vi "sub_DC Power End.vi"(8 "错误输入（无错误）":errorcluster, 10 "instrument handle out":refnum<k15>, 11 "IVI引用句柄输入":refnum<k15>) -> ()   [LabVIEW 2015]
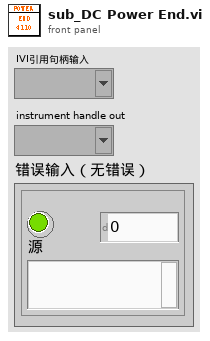
[diagram p1: front panel]
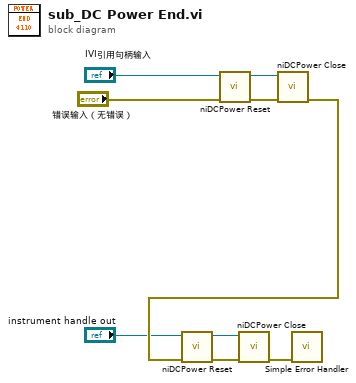
[diagram p0: block diagram]
diagram:
  n1 = call <instrlib>:"niDCPower Reset.vi"("error in (no error)"="错误输入（无错误）", "instrument handle"="IVI引用句柄输入") -> ("error out"=w3:errorcluster, "instrument handle out"=w2:refnum<k15>)  [unwired: 2 in, 6 out]
  n2 = call <instrlib>:"niDCPower Close.vi"("error in (no error)"=w3, "instrument handle"=w2) -> ("error out"=w9:errorcluster)  [unwired: 9 out]
  n3 = call <instrlib>:"niDCPower Reset.vi"("error in (no error)"=w9, "instrument handle"="instrument handle out") -> ("error out"=w5:errorcluster, "instrument handle out"=w6:refnum<k15>)  [unwired: 2 in, 6 out]
  n4 = call <instrlib>:"niDCPower Close.vi"("error in (no error)"=w5, "instrument handle"=w6) -> ("error out"=w4:errorcluster)  [unwired: 9 out]
  n5 = call <vilib>:"Simple Error Handler.vi"("error in (no error)"=w4) -> ()  [unwired: 1 in, 8 out]
